vi "Box Plot and Violin Plot Example.vi"() -> ()   [LabVIEW 2019]
uses:
  Python Visualizations Library/plot_labels.ctl
  Python Visualizations Library/Python Visualizations.lvlib
  <vilib>/Analysis/NI_AALBase.lvlib
panel:
  in  "Standard Deviation for\nGenerated Datasets":dbl[](array[numeric])=[6.0, 7.0, 8.0]
  out "Datasets":string[][](table)
  out "Violin Plot":picture
  out "Box Plot":picture
  in  "labels":T1={"dataset labels"=["A001", "A002", "B005"], "title"="DUT Results", "x-axis label"="DUT", "y-axis label"="Voltage (V)"}
  # "Generate Data"
  # "Data Visualizations"
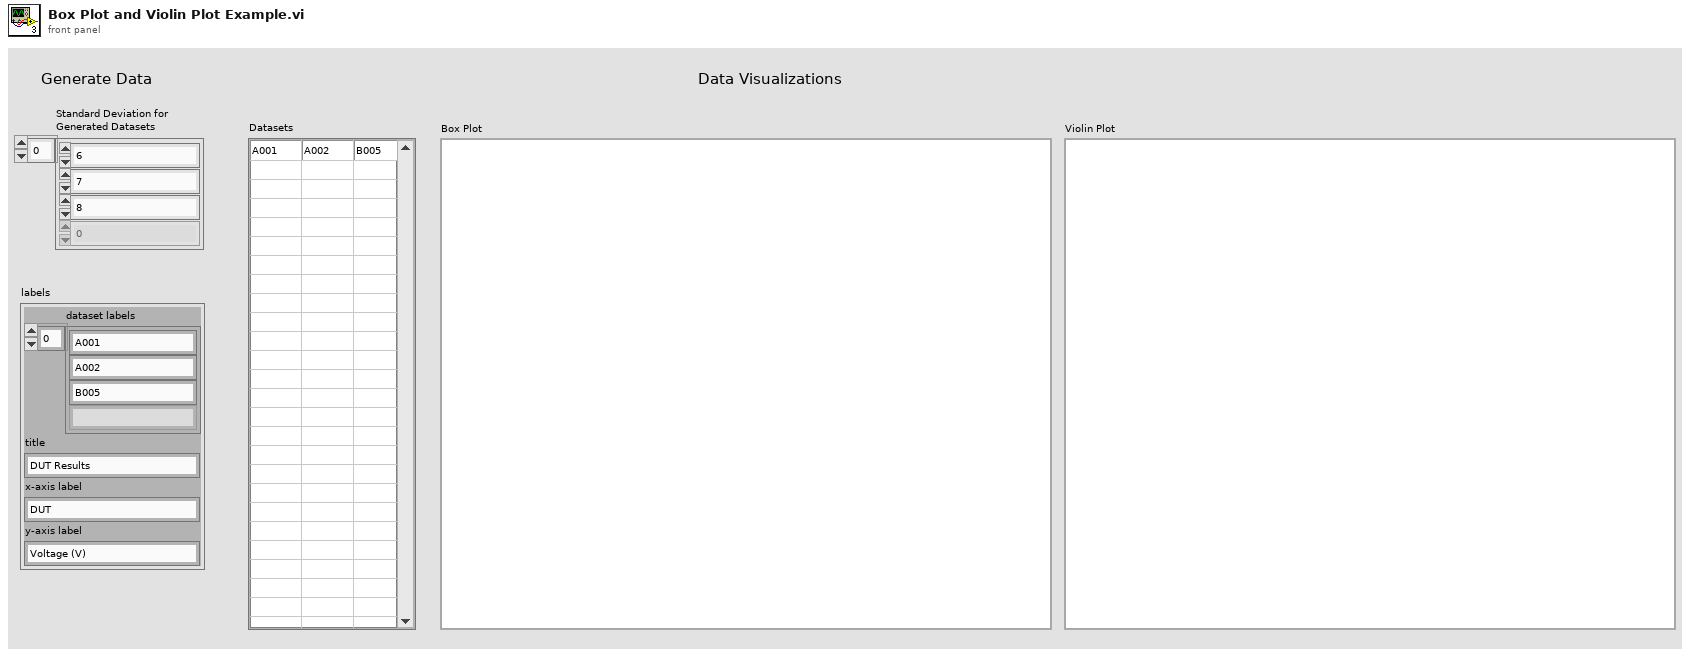
[diagram p1: front panel]
types:
  T1 = typedef "Python Visualizations.lvlib/plot_labels.ctl" = cluster{"dataset labels":string[], "title":string, "x-axis label":string, "y-axis label":string}
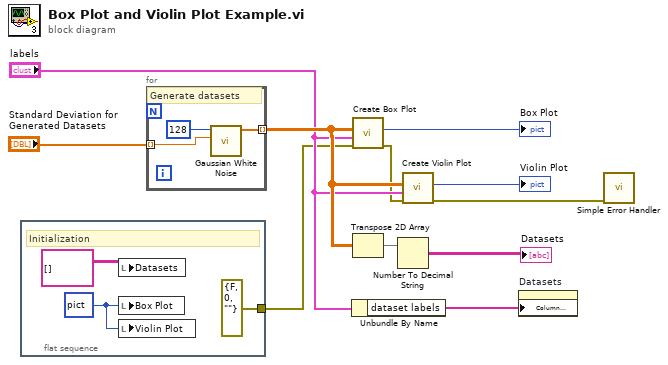
[diagram p0: block diagram]
diagram:
  n1 = flat-sequence {
    tunnel: [errorcluster {"status"=FALSE, "code"=0, "source"=""} ("error in (no error)")] -> w1
    frame #0 {
      w12 = picture data[5B] ("Box Plot")
      # "Initialization"
      n2 = local write "Datasets"(string[][] [] ("Datasets")) -> ()
      n3 = local write "Box Plot"(w12) -> ()
      n4 = local write "Violin Plot"(w12) -> ()
    }
  }
  n5 = for {
    tunnel: "Standard Deviation for\nGenerated Datasets" -> [w16] mode=indexing
    tunnel: [w15] -> w6 mode=indexing
    # "Generate datasets"
    n6 = call <vilib>:"Gaussian White Noise.vi"("standard deviation"=w16, "samples"=128) -> ("Gaussian noise pattern"=w15:dbl[])  [unwired: 8 in, 1 out]
  }
  n7 = Unbundle By Name("labels") -> ("dataset labels"=w4:string[])
  n8 = call "Create Box Plot.vi"("error in (no error)"=w1, "labels"="labels", "datasets"=w6) -> ("error out"=w3:errorcluster, "boxplot"=→"Box Plot":picture)  [unwired: 7 in]
  n9 = Transpose 2D Array(2D array=w6) -> (transposed array=w8:dbl[][])
  n10 = Number To Decimal String(number=w8) -> (decimal integer string=→"Datasets":string[][])  [unwired: 1 in]
  n11 = call "Create Violin Plot.vi"("error in (no error)"=w3, "labels"="labels", "datasets"=w6) -> ("error out"=w2:errorcluster, "violinplot"=→"Violin Plot":picture)  [unwired: 7 in]
  n12 = property on="Datasets" class="Tbl (strict)"("Column Headers[]"=w4) -> ()  [unwired: 2 in, 2 out]
  n13 = call <vilib>:"Simple Error Handler.vi"("error in (no error)"=w2) -> ()  [unwired: 4 in, 5 out]
